vi "Restart Sound.vi"(4 "error IN":errorcluster, 5 "sound format":T2, 6 "time (ms)":dbl, 7 "task ID IN":T1 format="%.0x") -> (0 "error OUT":errorcluster, 1 "#samples":u32, 3 "task ID OUT":T1 format="%.0x")   [LabVIEW 2010]
uses:
  <vilib>/sound2/lvsound2.llb/Sound Output Task ID.ctl
  <vilib>/sound2/lvsound2.llb/Sound Data Format.ctl
  <vilib>/sound2/lvsound2.llb/Sampling Mode.ctl
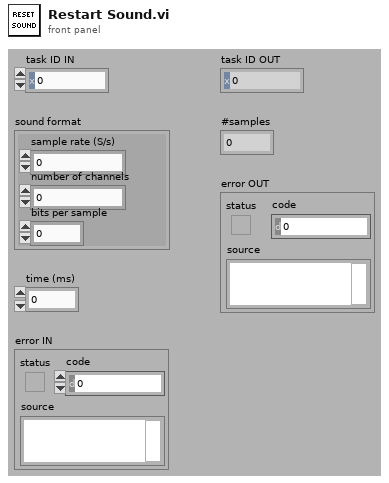
[diagram p1: front panel]
types:
  T1 = typedef "Sound Output Task ID.ctl" = u32
  T2 = typedef "Sound Data Format.ctl" = cluster{"sample rate (S/s)":dbl, "number of channels":i32, "bits per sample":i32}
  T3 = typedef "Sampling Mode.ctl" = i32
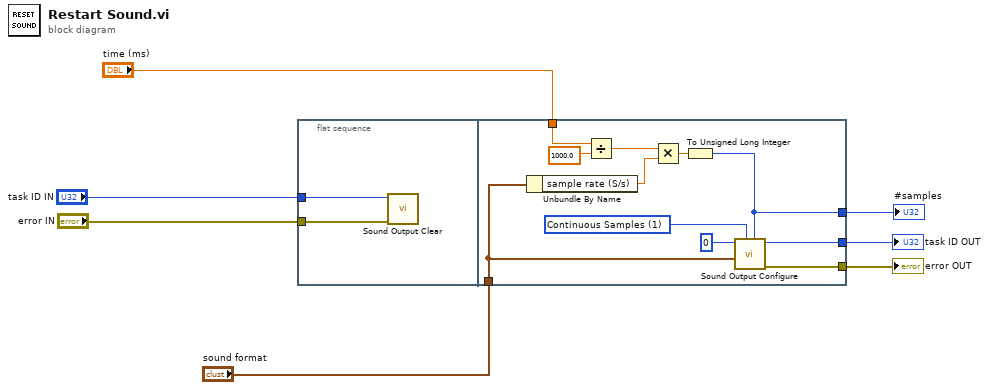
[diagram p0: block diagram]
diagram:
  n1 = flat-sequence {
    tunnel: "task ID IN" -> [w9]
    tunnel: "error IN" -> [w8]
    tunnel: [w14] -> w7
    tunnel: [w13] -> w6
    tunnel: [w12] -> w5
    tunnel: "time (ms)" -> [w11]
    tunnel: "sound format" -> [w10]
    frame #0 {
      n2 = call <vilib>:"Sound Output Clear.vi"("error in (no error)"=w8, "task ID"=w9) -> ()  [unwired: 9 in, 1 out]
    }
    frame #1 {
      w15 = T3 1 items=["Finite Samples", "Continuous Samples"] ("sample mode")
      n3 = Unbundle By Name(w10) -> ("sample rate (S/s)"=w17:dbl)
      n4 = Divide(x=w11, y=sgl 1000.0) -> (x/y=w18:dbl)
      n5 = Multiply(x=w18, y=w17) -> (x*y=w19:dbl)
      n6 = To Unsigned Long Integer(number=w19) -> (unsigned 32bit integer=w12:u32)
      n7 = call <vilib>:"Sound Output Configure.vi"("number of samples/ch"=w12, "sample mode"=w15, "sound format"=w10, "device ID"=u32 0) -> ("error out"=w13:errorcluster, "task ID"=w14:T1)  [unwired: 6 in]
    }
  }
  "#samples" <- w5
  "error OUT" <- w6
  "task ID OUT" <- w7
